vi "Teleop.vi"(10 "Match Info":T1={"Autonomous Elapsed Seconds"=0.0, "TeleOp Elapsed Seconds"=0.0, "Disabled Elapsed Seconds"=0.0, "Visited Autonomous"=FALSE, "Visited TeleOp"=FALSE, "Visited Disabled"=FALSE, "Autonomous Settings"={"Autonomous Style"=enum."Independent", "VI Refnum"=refnum}}, 11 "Call Context":T2) -> ()   [LabVIEW 2014]
doc: "This VI is called for each TeleOp packet received from the DS where the robot is not disabled. It is often used to read from the joysticks and update I/O or to update setpoints for timed control loops. It should complete and return within 20 milliseconds or it may miss DS packets."
uses:
  <vilib>/Rock Robotics/WPI/DriverStation/WPI_DriverStationDerivedRobotMode.ctl
  <vilib>/Rock Robotics/WPI/DriverStation/WPI_DriverStationMatch Info.ctl
  Robot Global Data.vi
  900/Team900-VIs/Logitech/F510/F510-X.vi
  <vilib>/Rock Robotics/Network Tables/SD Write Numeric Array.vi
  900/SwerveDrive/SwerveDriveFuse.vi
  <vilib>/Rock Robotics/WPI/DriverStation/WPI_DriverStationRobotMode2.ctl
  900/TeleArm/ArmControl.vi
  900/TeleArm/ArcadeArmControl.vi
panel:
  out "error out":errorcluster
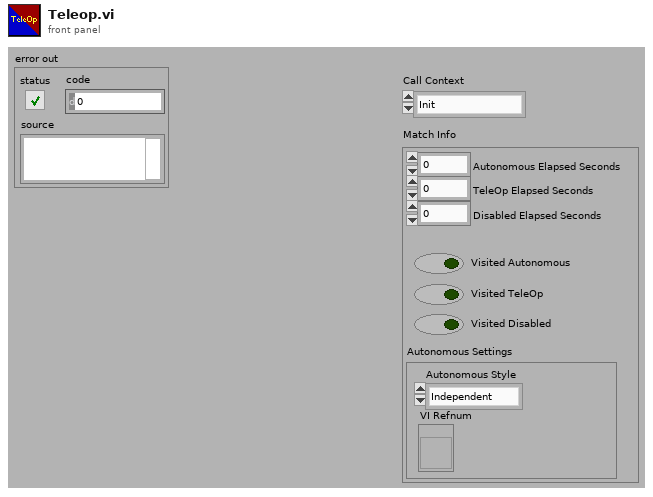
[diagram p1: front panel]
types:
  T1 = typedef "WPI_DriverStationMatch Info.ctl" = cluster{"Autonomous Elapsed Seconds":dbl, "TeleOp Elapsed Seconds":dbl, "Disabled Elapsed Seconds":dbl, "Visited Autonomous":bool, "Visited TeleOp":bool, "Visited Disabled":bool, "Autonomous Settings":cluster{"Autonomous Style":enum16{"Iterative", "Independent"}, "VI Refnum":refnum<vi>}}
  T2 = typedef "WPI_DriverStationDerivedRobotMode.ctl" = enum16{"Init", "Execute", "Stop"}
  T3 = cluster{"proportional gain (Kc)":dbl, "integral time (Ti, min)":dbl, "derivative time (Td, min)":dbl}
  T4 = cluster{"A":bool, "B":bool, "X":bool, "Y":bool, "LB":bool, "RB":bool, "Back":bool, "Start":bool, "LC":bool, "RC":bool, "LT":bool, "RT":bool}
  T5 = typedef "WPI_DriverStationRobotMode2.ctl" = enum16{"Autonomous Disabled", "Autonomous Enabled", "Teleop Disabled", "Teleop Enabled", "Disconnected", "Finish", "Test Disabled", "Test Enabled", "Emergency Stopped"}
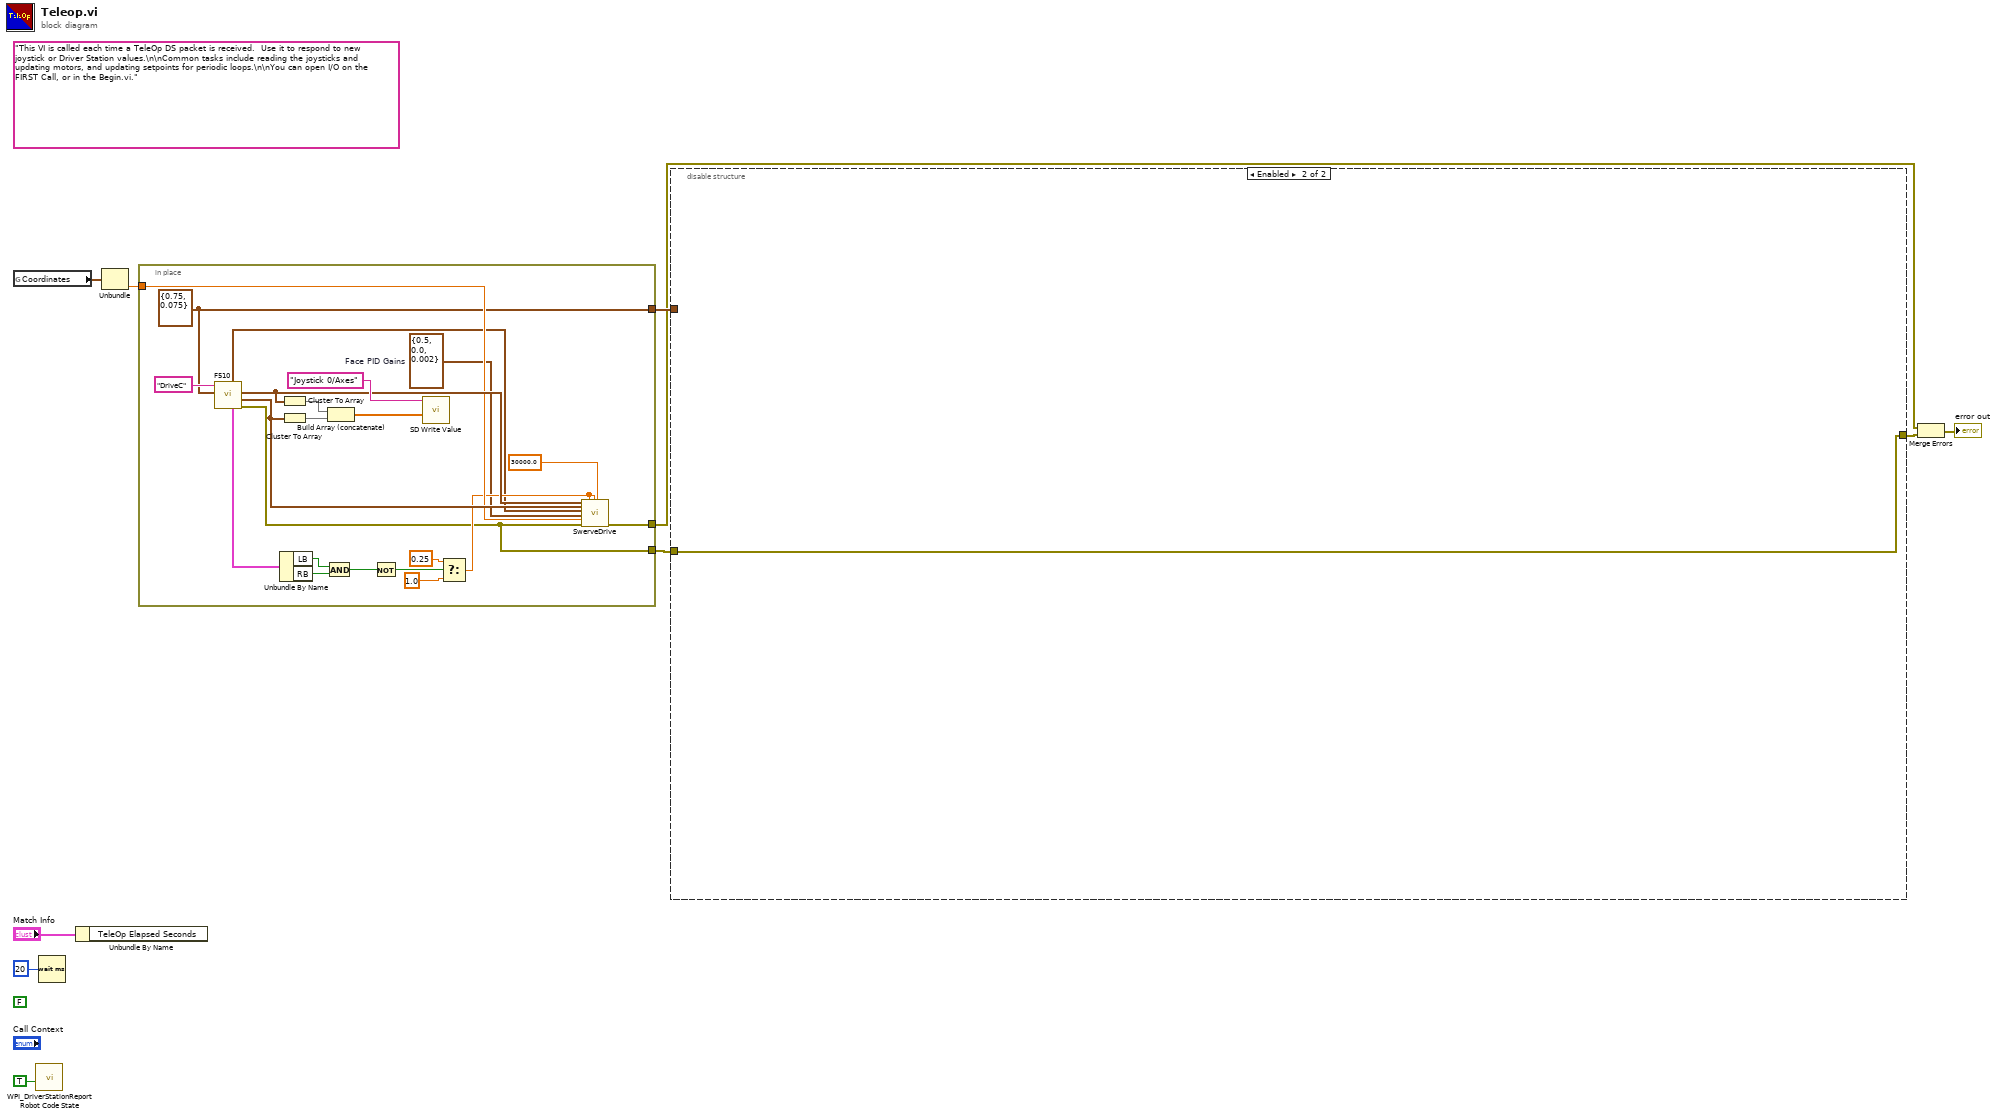
[diagram p0: block diagram]
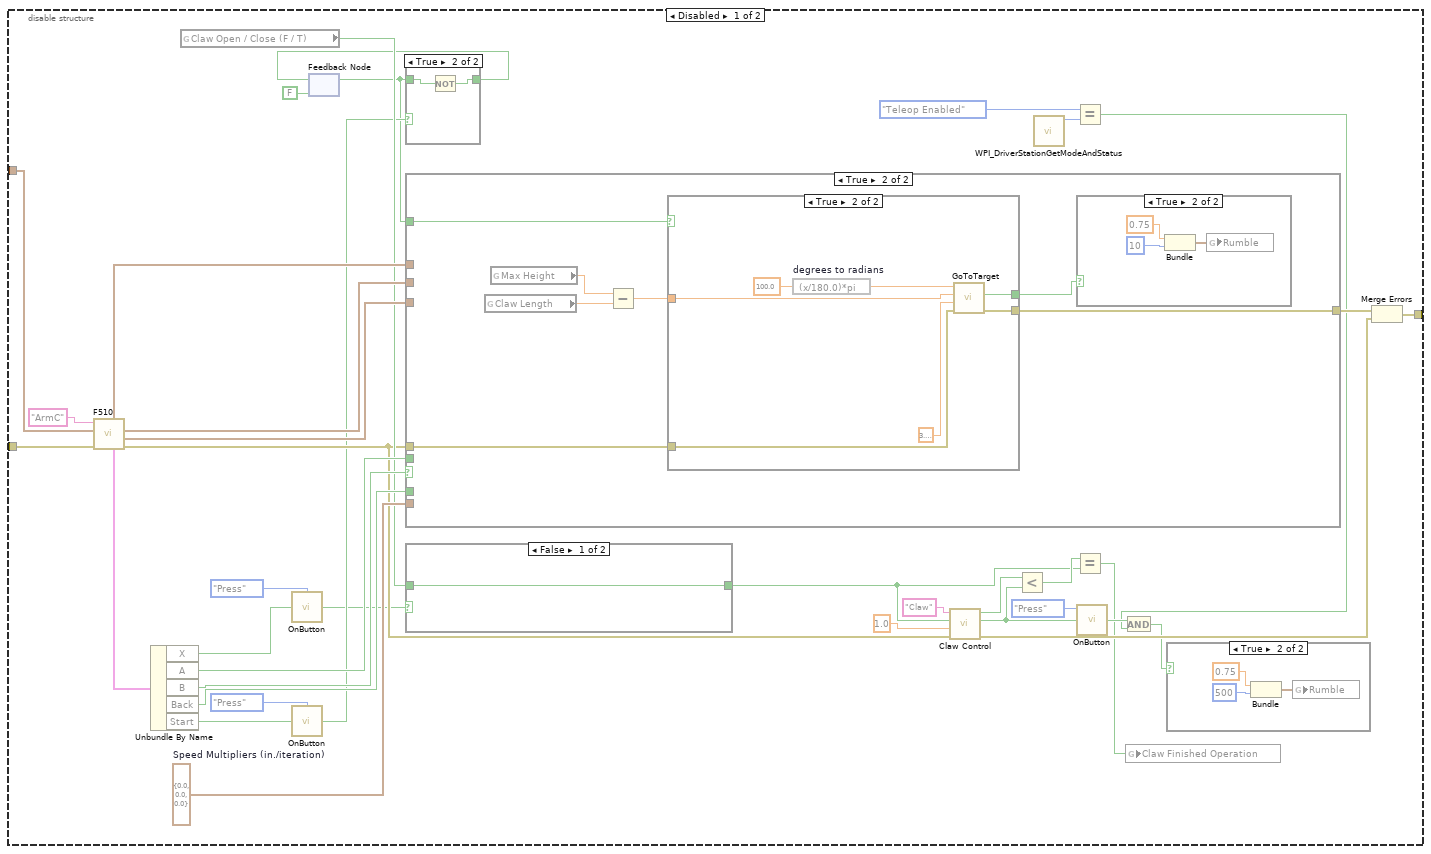
[diagram p2: hidden frame]
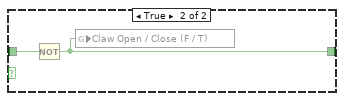
[diagram p4: hidden frame]
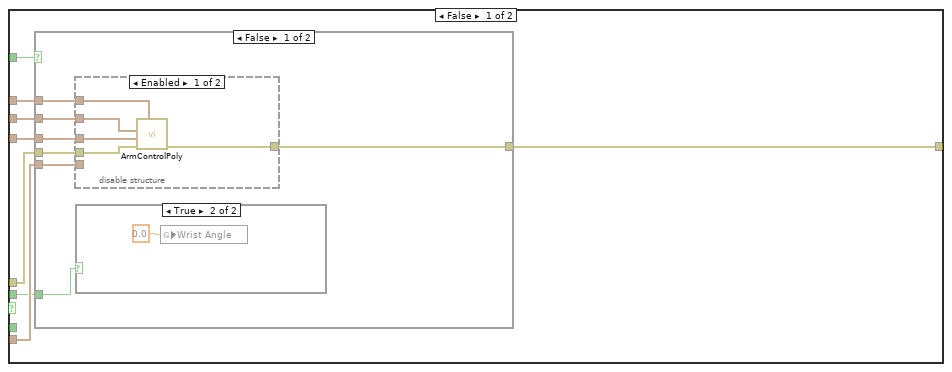
[diagram p6: hidden frame]
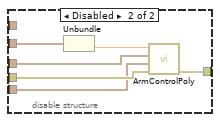
[diagram p8: hidden frame]
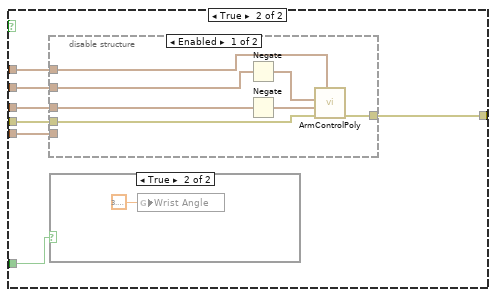
[diagram p9: hidden frame]
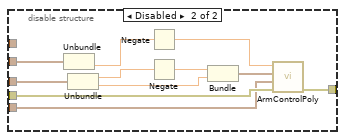
[diagram p11: hidden frame]
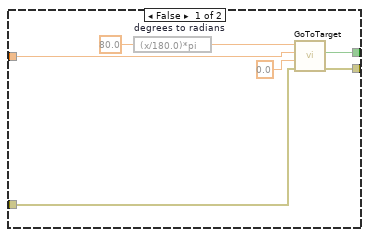
[diagram p13: hidden frame]
diagram:
  (unwired) FALSE
  (unwired) "This VI is called each time a TeleOp DS packet is received.  Use it to respond to new joystick or Driver Station values.\n\nCommon tasks include reading the joysticks and updating motors, and updating setpoints for periodic loops.\n\nYou can open I/O on the FIRST Call, or in the Begin.vi."
  n1 = global read "Robot Global Data.vi" "Coordinates"() -> (w1:cluster{"X":dbl, "Y":dbl, "Heading":dbl})
  n2 = call <vilib>:"WPI_DriverStationReport Robot Code State.vi"("TeleOp"=TRUE ("Autonomous")) -> ()  [unwired: 10 in, 1 out]
  n3 = Wait (ms)(milliseconds to wait=u32 20) -> ()  [unwired: 1 out]
  n4 = Unbundle By Name("Match Info") -> ()  [unwired: 1 out]
  n5 = Unbundle(w1) -> ("Heading"=w2:dbl)  [unwired: 2 out]
  n6 = in-place {
    in-place-border: w2 -> [w21]
    in-place-border: [w14] -> w8
    in-place-border: [w13] -> w6
    in-place-border: [w12] -> w3
    w15 = T3 {"proportional gain (Kc)"=0.5, "integral time (Ti, min)"=0.0, "derivative time (Td, min)"=0.002}  # Face PID Gains
    w13 = cluster{"Scale":dbl, "Deadzone":dbl} {"Scale"=0.75, "Deadzone"=0.075} ("Deadzone Scale Cluster")
    n7 = call-poly "F510.vi"("Deadzone Scale Cluster"=w13, "refnum name"="DriveC") -> ("error out"=w14:errorcluster, "Right Stick"=w30:cluster{"X":dbl, "Y":dbl}, "Left Stick"=w31:cluster{"X":dbl, "Y":dbl}, "Buttons"=w23:T4, "Triggers"=w11:cluster{"Left":dbl, "Right":dbl})  [unwired: 3 in, 2 out]
    n8 = Unbundle By Name(w23) -> ("LB"=w25:bool, "RB"=w24:bool)
    n9 = Cluster To Array(cluster=w31) -> (array=w29:dbl[])
    n10 = Cluster To Array(cluster=w30) -> (array=w28:dbl[])
    n11 = And(x=w25, y=w24) -> (x .and. y?=w26:bool)
    n12 = Build Array (concatenate)(w29, w28) -> (w27:dbl[])
    n13 = Not(x=w26) -> (.not. x?=w17:bool)
    n14 = call-poly <vilib>:"SD Write Value.vi"("Numeric Array"=w27, "Name"="Joystick 0/Axes") -> ()  [unwired: 8 in, 2 out]
    n15 = Select(t=0.25 ("Slow Speed Multiplier"), s=w17, f=1.0 ("Default Speed Multiplier")) -> (s? t:f=w16:dbl)
    n16 = call-poly "SwerveDrive.vi"("Strafe Joystick Axes"=w31, "Face Joystick Axes"=w30, "Trigger Axes"=w11, "Face PID Gains"=w15, "Angle (degrees; 0 = right)"=w21, "error in (no error)"=w14, "Strafe Multiplier"=w16, "Rotation Multiplier"=w16, "Max Wheel Speed"=30000.0 ("Default Speed Multiplier")) -> ("error out"=w12:errorcluster)  [unwired: 10 in]
  }
  n17 = disable-structure shown="Enabled" {
    disable-tunnel: w8 -> [w69 w157]
    disable-tunnel: w6 -> [w34 _]
    disable-tunnel: [w33 w157] -> w5
    frame Disabled {
      w61 = cluster{"X":dbl, "Y":dbl, "Wrist":dbl} {"X"=0.0, "Y"=0.0, "Wrist"=0.0}  # Speed Multipliers (in./iteration)
      n18 = call-poly "F510.vi"("error in (no error)"=w69, "Deadzone Scale Cluster"=w34, "refnum name"="ArmC") -> ("error out"=w58:errorcluster, "Right Stick"=w65:cluster{"X":dbl, "Y":dbl}, "Left Stick"=w66:cluster{"X":dbl, "Y":dbl}, "Buttons"=w68:T4, "Triggers"=w67:cluster{"Left":dbl, "Right":dbl})  [unwired: 2 in, 2 out]
      n19 = Unbundle By Name(w68) -> ("X"=w48:bool, "A"=w62:bool, "B"=w63:bool, "Back"=w64:bool, "Start"=w51:bool)
      n20 = global read "Robot Global Data.vi" "Claw Open / Close (F / T)"() -> (w60:bool)
      n21 = call "OnButton.vi"("Button"=w48, "Mode"=enum16{"Press", "Release", "Both"}."Press") -> ("Value"=w47:bool)
      n22 = call "OnButton.vi"("Button"=w51, "Mode"=enum16{"Press", "Release", "Both"}."Press") -> ("Value"=w50:bool)
      n23 = feedback #1(FALSE) -> (w36:bool)
      n24 = case shown="True" w50 {
        tunnel: [w77 w79] -> w37
        tunnel: w36 -> [w77 w78]
        frame False {
        }
        frame True {
          n25 = Not(x=w78) -> (.not. x?=w79:bool)
        }
      }
      n26 = feedback-in #1(w37) -> ()
      n27 = case shown="True" w63 {
        tunnel: [w82 w138] -> w56
        tunnel: w67 -> [w86 _]
        tunnel: w66 -> [w87 _]
        tunnel: w65 -> [w85 _]
        tunnel: w58 -> [w84 w139]
        tunnel: w36 -> [w81 w134]
        tunnel: w64 -> [_ _]
        tunnel: w61 -> [w83 _]
        tunnel: w62 -> [w80 _]
        frame False {
          n28 = case shown="False" w81 {
            tunnel: w87 -> [w90 w113]
            tunnel: w86 -> [w89 w112]
            tunnel: w85 -> [w91 w111]
            tunnel: w84 -> [w94 w110]
            tunnel: w83 -> [w92 w109]
            tunnel: [w93 w108] -> w82
            tunnel: w80 -> [w88 w107]
            frame False {
              n29 = disable-structure shown="Enabled" {
                disable-tunnel: [w100 w105] -> w93
                disable-tunnel: w89 -> [w99 _]
                disable-tunnel: w90 -> [w97 w103]
                disable-tunnel: w91 -> [w96 w104]
                disable-tunnel: w94 -> [w98 w106]
                disable-tunnel: w92 -> [_ w101]
                frame Enabled {
                  n30 = call-poly "ArmControlPoly.vi"("Extension Triggers"=w99, "error in (no error)"=w98, "Pivot Stick"=w96, "Wrist Stick"=w97) -> ("error out"=w100:errorcluster)  [unwired: 7 in]
                }
                frame Disabled {
                  n31 = Unbundle(w103) -> ("Y"=w102:dbl)  [unwired: 1 out]
                  n32 = call-poly "ArmControlPoly.vi"("error in (no error)"=w106, "Speed Multipliers"=w101, "X/Y Stick"=w104, "Wrist rotation (radians/iteration)"=w102) -> ("error out"=w105:errorcluster)  [unwired: 7 in]
                }
              }
              n33 = case shown="True" w88 {
                frame False {
                }
                frame True {
                  n34 = global write "Robot Global Data.vi" "Wrist Angle"(0.0 ("Wrist Angle")) -> ()
                }
              }
            }
            frame True {
              n35 = disable-structure shown="Enabled" {
                disable-tunnel: [w121 w131] -> w108
                disable-tunnel: w112 -> [w120 _]
                disable-tunnel: w113 -> [w118 w130]
                disable-tunnel: w111 -> [w117 w127]
                disable-tunnel: w110 -> [w119 w132]
                disable-tunnel: w109 -> [_ w128]
                frame Enabled {
                  n36 = Negate(x=w118) -> (-x=w116:cluster{"X":dbl, "Y":dbl})
                  n37 = Negate(x=w117) -> (-x=w115:cluster{"X":dbl, "Y":dbl})
                  n38 = call-poly "ArmControlPoly.vi"("Extension Triggers"=w120, "error in (no error)"=w119, "Pivot Stick"=w115, "Wrist Stick"=w116) -> ("error out"=w121:errorcluster)  [unwired: 7 in]
                }
                frame Disabled {
                  n39 = Unbundle(w130) -> ("Y"=w129:dbl)  [unwired: 1 out]
                  n40 = Unbundle(w127) -> ("X"=w125:dbl, "Y"=w126:dbl)
                  n41 = Negate(x=w129) -> (-x=w122:dbl)
                  n42 = Negate(x=w125) -> (-x=w124:dbl)
                  n43 = Bundle(w124, "Y"=w126) -> (w123:cluster{dbl, "Y":dbl})  [unwired: 1 in]
                  n44 = call-poly "ArmControlPoly.vi"("error in (no error)"=w132, "Speed Multipliers"=w128, "X/Y Stick"=w123, "Wrist rotation (radians/iteration)"=w122) -> ("error out"=w131:errorcluster)  [unwired: 7 in]
                }
              }
              n45 = case shown="True" w107 {
                frame False {
                }
                frame True {
                  n46 = global write "Robot Global Data.vi" "Wrist Angle"(3.141592653589793) -> ()
                }
              }
            }
          }
        }
        frame True {
          n47 = global read "Robot Global Data.vi" "Claw Length"() -> (w136:dbl)
          n48 = global read "Robot Global Data.vi" "Max Height"() -> (w137:dbl)
          n49 = Subtract(x=w137, y=w136) -> (x-y=w135:dbl)
          n50 = case shown="True" w134 {
            tunnel: w139 -> [w148 w155]
            tunnel: [w149 w156] -> w138
            tunnel: w135 -> [w145 w151]
            tunnel: [w143 w150] -> w133
            frame False {
              n51 = expression code="(x/180.0)*pi" "degrees to radians"(80.0 ("target arm angle (rad)")) -> (w146:dbl)
              n52 = call "GoToTarget.vi"("error in (no error)"=w148, "target wrist angle (rad; relative to ground)"=0.0, "target extension (in.)"=w145, "target arm angle (rad)"=w146) -> ("error out"=w149:errorcluster, "finished"=w143:bool)  [unwired: 6 in]
            }
            frame True {
              n53 = expression code="(x/180.0)*pi" "degrees to radians"(100.0 ("target arm angle (rad)")) -> (w153:dbl)
              n54 = call "GoToTarget.vi"("error in (no error)"=w155, "target wrist angle (rad; relative to ground)"=3.141592653589793, "target extension (in.)"=w151, "target arm angle (rad)"=w153) -> ("error out"=w156:errorcluster, "finished"=w150:bool)  [unwired: 6 in]
            }
          }
          n55 = case shown="True" w133 {
            frame False {
            }
            frame True {
              n56 = Bundle("t"=0.75, "f"=i16 10) -> (w140:cluster{"t":dbl, "f":i16})  [unwired: 1 in]
              n57 = global write "Robot Global Data.vi" "Rumble"(w140) -> ()
            }
          }
        }
      }
      n58 = case shown="False" w47 {
        tunnel: [w74 w75] -> w43
        tunnel: w60 -> [w74 w76]
        frame False {
        }
        frame True {
          n59 = Not(x=w76) -> (.not. x?=w75:bool)
          n60 = global write "Robot Global Data.vi" "Claw Open / Close (F / T)"(w75) -> ()
        }
      }
      n61 = call "Claw Control.vi"("error in (no error)"=w58, "Output"=1.0, "Open / Close (F / T)"=w43, "Motor Name"="Claw") -> ("error out"=w55:errorcluster, "Closed"=w46:bool, "Open"=w45:bool)  [unwired: 3 in]
      n62 = Less?(x=w45, y=w46) -> (x < y?=w44:bool)
      n63 = call <vilib>:"WPI_DriverStationGetModeAndStatus.vi"() -> ("Robot Mode"=w40:T5)  [unwired: 10 in, 1 out]
      n64 = Equal?(x=WPI_DriverStationRobotMode2."Teleop Enabled", y=w40) -> (x = y?=w38:bool)
      n65 = Equal?(x=w44, y=w43) -> (x = y?=w42:bool)
      n66 = call "OnButton.vi"("Button"=w46, "Mode"=enum16{"Press", "Release", "Both"}."Press") -> ("Value"=w53:bool)
      n67 = And(x=w53, y=w38) -> (x .and. y?=w41:bool)
      n68 = global write "Robot Global Data.vi" "Claw Finished Operation"(w42) -> ()
      n69 = case shown="True" w41 {
        frame False {
        }
        frame True {
          n70 = Bundle("t"=0.75, "f"=i16 500) -> (w71:cluster{"t":dbl, "f":i16})  [unwired: 1 in]
          n71 = global write "Robot Global Data.vi" "Rumble"(w71) -> ()
        }
      }
      n72 = Merge Errors(w56, w55) -> (w33:errorcluster)
    }
    frame Enabled {
    }
  }
  n73 = Merge Errors(w3, w5) -> (→"error out":errorcluster)
